vi "solar_write SOLARUE_MSG.vi"(8 "error in (no error)":errorcluster, 10 "MESSAGE":cluster{"MSG":string, "DATA":variant}, 11 "solar in":refnum<class "solar.lvclass">) -> (0 "error out":errorcluster, 3 "solar out":refnum<class "solar.lvclass">)   [LabVIEW 2018, in "solar.lvclass"]
doc: "This writes a message to the SOLAR user interface user event."
uses:
  solar.lvclass
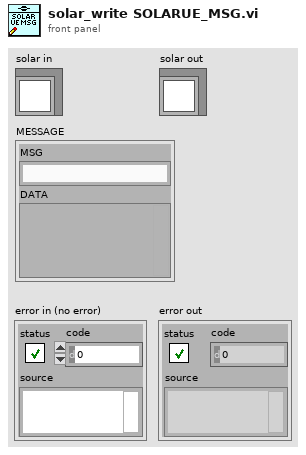
[diagram p1: front panel]
types:
  T1 = typedef "solar_ctl SOLAR Refnum.ctl" = refnum<k1>
  T2 = typedef "solar_ctl SOLAR Global.ctl" = cluster{"Targets":T3[], "AppDir":path, "solar.ini":path, "ConfigsDir":path, "CosmosDir":path, "LogsDir":path, "ExePath":path, "ExeVersion":string, "PartNum":string, "AppSetup":string, "Title":string, "Main.ini":path, "Temp.ini":path, "vSOLAR":string, "Splash.png":string, "SplashWait":i32, "SOLARUE":refnum<user-event>, "VoyagerRefnum":T4, "QTimerRefnum":T5}
  T3 = typedef "solar_ctl Target Global.ctl" = cluster{"Target":string, "Q":refnum<queue>, "UE":refnum<user-event>, "VI":refnum<vi>, "Menu":refnum<k9>, "Data":refnum<data-value>, "Attributes":variant}
  T4 = typedef "solar_voy_ctl Voyager Refnum.ctl" = refnum<k1>
  T5 = typedef "solar_qtimer_ctl Refnum.ctl" = refnum<k1>
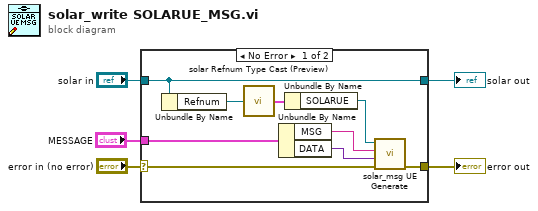
[diagram p0: block diagram]
diagram:
  n1 = case shown="No Error" "error in (no error)" {
    selector: "error in (no error)" -> [w11 w16]
    tunnel: "solar in" -> [w12 w15]
    tunnel: [w10 w16] -> w4
    tunnel: [w12 w15] -> w2
    tunnel: "MESSAGE" -> [w8 _]
    frame No Error {
      n2 = Unbundle By Name(w12) -> ("Refnum"=w14:T1)
      n3 = call "solar Refnum Type Cast (Preview).vi"("Refnum"=w14) -> ("SOLAR"=w13:T2)  [unwired: 8 in]
      n4 = Unbundle By Name(w8) -> ("MSG"=w7:string, "DATA"=w6:variant)
      n5 = Unbundle By Name(w13) -> ("SOLARUE"=w9:refnum<user-event>)
      n6 = call "solar_msg UE Generate.vi"("error in (no error)"=w11, "CMD_DATA (Last)"=w6, "CMD (Last)"=w7, "UserEvent in"=w9) -> ("error out"=w10:errorcluster)  [unwired: 6 in, 1 out]
    }
    frame Error {
    }
  }
  "error out" <- w4
  "solar out" <- w2
